vi "TestItemsIndex.vi"(4 "semaphore":T1 caption="信号量", 6 "TestItemIndexIn":i32, 8 "ErrorIn(NoError)":errorcluster, 9 "GuiRef":T2={"StringOut"=refnum, "AbortOnFail"=refnum, "SN"=refnum, "SN_Length"=refnum, "TestResult"=refnum, "CycleTime"=refnum, "ErrorCode"=refnum, "UUTStatus"=refnum, "DataBaseEnable?"=refnum, "DUTModel"=refnum, "FixtureID"=refnum, "OperatorID"=refnum, "SNReady"=refnum, "StopSlot"=refnum, "NextStep"=refnum, "PassYeild"=refnum, "Failed"=refnum, "Passed"=refnum, "Tested"=refnum, "TestItemsCtl"={"StepName"="", "TestEnable"=FALSE, "LoopCount"=0, "StopOnFail"=FALSE, "Index"=0, "TestName"="", "通道"="", "参数"="", "TimeStart"=0}, "ProcessBar"=refnum, "Slot"=enum."Slot1", "Row"=3, "States"=refnum, "TestMode"=refnum, "循环次数-DUT"=refnum, "波形图"=refnum, "产品型号"=refnum, "子面板"=refnum, "测试失败项目"=refnum, "测试结果"=refnum, "DUT"=refnum, "Starttime"=refnum, "SlotReady"=refnum, "版本信息"=refnum, "WIFI_1"=refnum, "WIFI_2"=refnum, "直通率"=refnum, "卡1开卡结果"=refnum, "卡2开卡结果"=refnum}, 11 "Fail项目":string[](array[string])) -> (0 "ErrorOut":errorcluster, 1 "GuiRefOut":T2={"StringOut"=refnum, "AbortOnFail"=refnum, "SN"=refnum, "SN_Length"=refnum, "TestResult"=refnum, "CycleTime"=refnum, "ErrorCode"=refnum, "UUTStatus"=refnum, "DataBaseEnable?"=refnum, "DUTModel"=refnum, "FixtureID"=refnum, "OperatorID"=refnum, "SNReady"=refnum, "StopSlot"=refnum, "NextStep"=refnum, "PassYeild"=refnum, "Failed"=refnum, "Passed"=refnum, "Tested"=refnum, "TestItemsCtl"={"StepName"="", "TestEnable"=FALSE, "LoopCount"=0, "StopOnFail"=FALSE, "Index"=0, "TestName"="", "通道"="", "参数"="", "TimeStart"=0}, "ProcessBar"=refnum, "Slot"=enum."Slot1", "Row"=3, "States"=refnum, "TestMode"=refnum, "循环次数-DUT"=refnum, "波形图"=refnum, "产品型号"=refnum, "子面板"=refnum, "测试失败项目"=refnum, "测试结果"=refnum, "DUT"=refnum, "Starttime"=refnum, "SlotReady"=refnum, "版本信息"=refnum, "WIFI_1"=refnum, "WIFI_2"=refnum, "直通率"=refnum, "卡1开卡结果"=refnum, "卡2开卡结果"=refnum})   [LabVIEW 2013]
uses:
  SysControl/Reference.ctl
  SysControl/TestItemsCTL.ctl
  SysControl/Slot.ctl
  SourceCode/GlobalValue.vi
panel:
  out "Item Names":string[][](array[string])
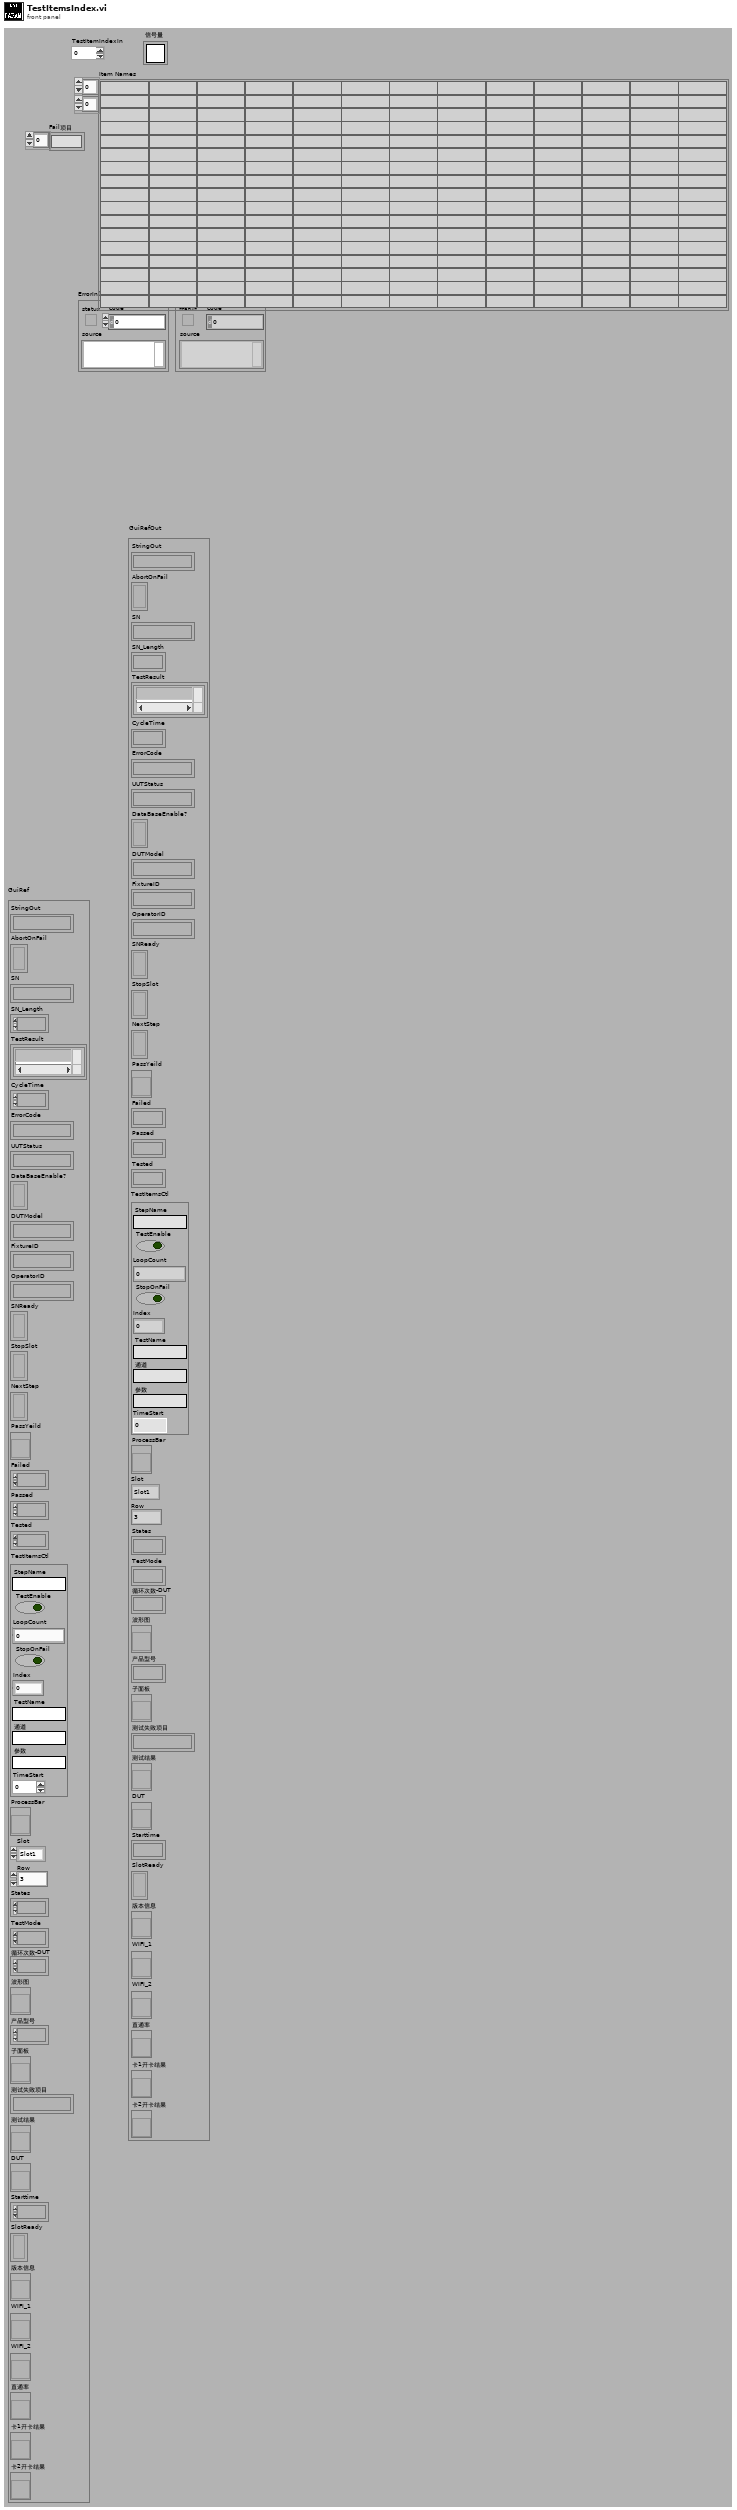
[diagram p1: front panel]
types:
  T1 = typedef "Semaphore RefNum" = refnum<k1>
  T2 = typedef "Reference.ctl" = cluster{"StringOut":refnum<vi>, "AbortOnFail":refnum<vi>, "SN":refnum<vi>, "SN_Length":refnum<vi>, "TestResult":refnum<vi>, "CycleTime":refnum<vi>, "ErrorCode":refnum<vi>, "UUTStatus":refnum<vi>, "DataBaseEnable?":refnum<vi>, "DUTModel":refnum<vi>, "FixtureID":refnum<vi>, "OperatorID":refnum<vi>, "SNReady":refnum<vi>, "StopSlot":refnum<vi>, "NextStep":refnum<vi>, "PassYeild":refnum<vi>, "Failed":refnum<vi>, "Passed":refnum<vi>, "Tested":refnum<vi>, "TestItemsCtl":T3, "ProcessBar":refnum<vi>, "Slot":T4, "Row":u32, "States":refnum<vi>, "TestMode":refnum<vi>, "循环次数-DUT":refnum<vi>, "波形图":refnum<vi>, "产品型号":refnum<vi>, "子面板":refnum<vi>, "测试失败项目":refnum<vi>, "测试结果":refnum<vi>, "DUT":refnum<vi>, "Starttime":refnum<vi>, "SlotReady":refnum<vi>, "版本信息":refnum<vi>, "WIFI_1":refnum<vi>, "WIFI_2":refnum<vi>, "直通率":refnum<vi>, "卡1开卡结果":refnum<vi>, "卡2开卡结果":refnum<vi>}
  T3 = typedef "TestItemsCTL.ctl" = cluster{"StepName":string, "TestEnable":bool, "LoopCount":i32, "StopOnFail":bool, "Index":u32, "TestName":string, "通道":string, "参数":string, "TimeStart":u32}
  T4 = typedef "Slot.ctl" = enum16{"Slot1", "Slot2", "Slot3", "Slot4"}
  T5 = enum16{"Production Mode", "Selection Mode", "Debug Mode", "Loop Mode", "Stop Test"}
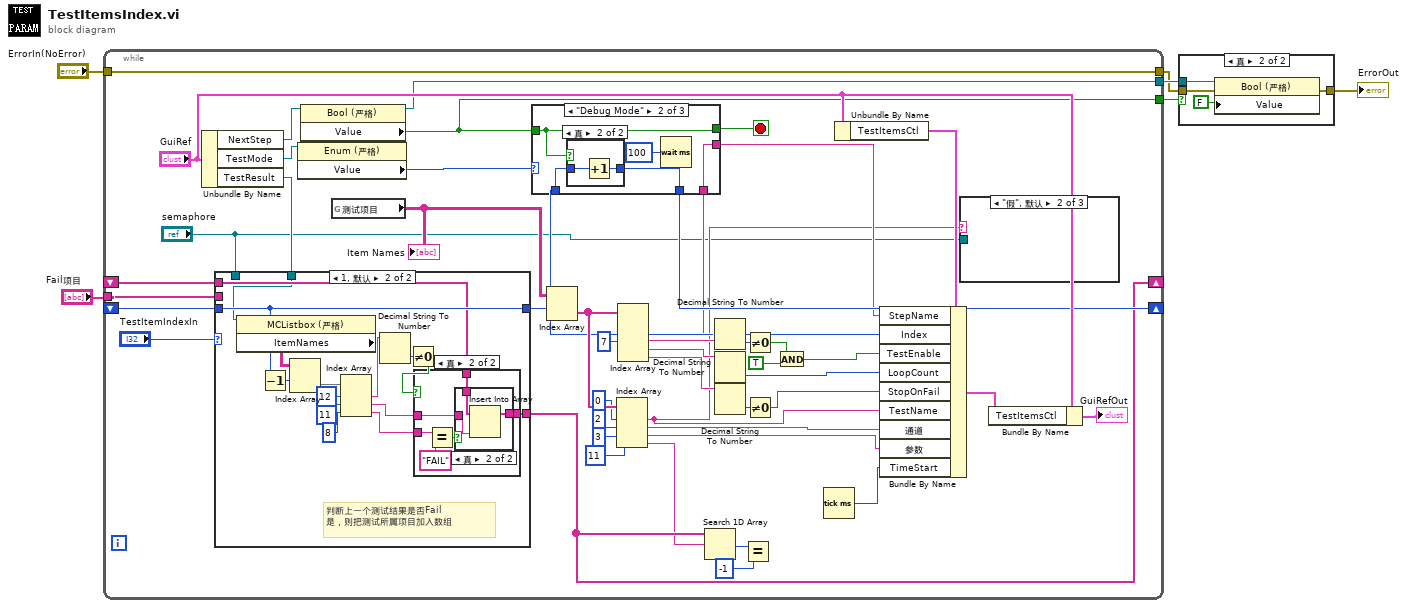
[diagram p0: block diagram]
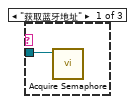
[diagram p3: hidden frame]
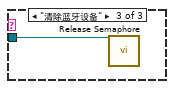
[diagram p4: hidden frame]
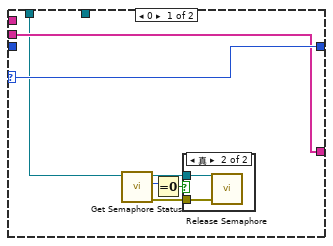
[diagram p5: hidden frame]
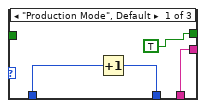
[diagram p9: hidden frame]
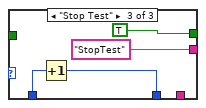
[diagram p11: hidden frame]
diagram:
  n1 = while {
    tunnel: "ErrorIn(NoError)" -> [w41]
    tunnel: [w41] -> w4
    shift-right: [w33] -> _
    shift-left: _ -> [w16]
    tunnel: [w32] -> w5
    tunnel: [w31] -> w3
    shift-right: [w25] -> _
    shift-left: _ -> [w19]
    tunnel: "Fail项目" -> [w20]
    stop <- w10 stop-if-true
    n2 = Unbundle By Name("GuiRef") -> ("NextStep"=w36:refnum<vi>, "TestMode"=w35:refnum<vi>, "TestResult"=w18:refnum<vi>)
    n3 = case shown="1, 默认" "TestItemIndexIn" {
      selector: "TestItemIndexIn" -> [w61 _]
      tunnel: [w61 w76] -> w26
      tunnel: w16 -> [_ w76]
      tunnel: [w60 w75] -> w25
      tunnel: w20 -> [w60 _]
      tunnel: w19 -> [_ w74]
      tunnel: w18 -> [_ w73]
      tunnel: "semaphore" -> [w55 _]
      frame 0 {
        n4 = call <vilib>:"Get Semaphore Status.vi"("semaphore"=w55) -> ("error out"=w57:errorcluster, "# available"=w59:i32, "semaphore out"=w58:T1)  [unwired: 5 in, 3 out]
        n5 = Equal To 0?(x=w59) -> (x = 0?=w56:bool)
        n6 = case shown="真" w56 {
          tunnel: w58 -> [_ w62]
          tunnel: w57 -> [_ w63]
          frame False {
          }
          frame True {
            n7 = call <vilib>:"Release Semaphore.vi"("error in (no error)"=w63, "semaphore"=w62) -> ()  [unwired: 4 in, 2 out]
          }
        }
      }
      frame 1, Default {
        # "判断上一个测试结果是否Fail\n是，则把测试所属项目加入数组"
        n8 = property class="MCListbox (严格)"(reference=w73) -> ("ItemNames"=w72:string[][])  [unwired: 1 in, 2 out]
        n9 = Decrement(x=w76) -> (x-1=w78:i32)
        n10 = Index Array(array=w72, index (row)=w78) -> (element=w77:string[])  [unwired: 1 in]
        n11 = Index Array(array=w77, index #1=12 ("索引"), index #2=11 ("索引"), index #3=8 ("索引")) -> (element #1=w65:string, element #2=w68:string, element #3=w67:string)
        n12 = Decimal String To Number(string=w65) -> (number=w66:i32)  [unwired: 3 out]
        n13 = Not Equal To 0?(x=w66) -> (x != 0?=w64:bool)
        n14 = case shown="真" w64 {
          tunnel: [w79 w83] -> w75
          tunnel: w74 -> [w79 w82]
          tunnel: w68 -> [_ w81]
          tunnel: w67 -> [_ w80]
          frame False {
          }
          frame True {
            n15 = Equal?(x=w80, y="FAIL") -> (x = y?=w85:bool)
            n16 = case shown="真" w85 {
              tunnel: w81 -> [_ w89]
              tunnel: [w86 w88] -> w83
              tunnel: w82 -> [w86 w87]
              frame False {
              }
              frame True {
                n17 = Insert Into Array(array=w87, new element=w89) -> (w88:string[])  [unwired: 1 in]
              }
            }
          }
        }
      }
    }
    n18 = property class="Enum (严格)"(reference=w35) -> ("Value"=w34:T5)  [unwired: 1 in, 2 out]
    n19 = property class="Bool (严格)"(reference=w36) -> (reference out=w32:refnum<vi>, "Value"=w31:bool)  [unwired: 1 in, 1 out]
    n20 = global read "GlobalValue.vi" "测试项目"() -> (w17:string[][])
    "Item Names" <- w17
    n21 = Index Array(array=w17, index (row)=w26) -> (element=w48:string[])  [unwired: 1 in]
    n22 = Index Array(array=w48, index #1=0 ("索引"), index #2=2 ("索引"), index #3=3 ("索引"), index #4=11 ("索引")) -> (element #1=w9:string, element #2=w47:string, element #3=w46:string, element #4=w12:string)
    n23 = Index Array(array=w48, index #3=7 ("index")) -> (element #2=w14:string, element #3=w45:string, element #4=w44:string, element #5=w43:string)  [unwired: 4 in, 1 out]
    n24 = case shown="\"Debug Mode\"" w34 {
      tunnel: w31 -> [_ w95 _]
      tunnel: w26 -> [w93 w98 w105]
      tunnel: [w92 w97 w104] -> w33
      tunnel: [TRUE w95 TRUE] -> w10
      tunnel: w14 -> [w91 w94 _]
      tunnel: [w91 w94 "StopTest" ("element")] -> w11
      frame "Production Mode", Default {
        n25 = Increment(x=w93) -> (x+1=w92:i32)
      }
      frame "Debug Mode" {
        n26 = case shown="真" w95 {
          tunnel: w98 -> [w99 w101]
          tunnel: [w99 w100] -> w97
          frame False {
          }
          frame True {
            n27 = Increment(x=w101) -> (x+1=w100:i32)
          }
        }
        n28 = Wait (ms)(milliseconds to wait=u32 100) -> ()  [unwired: 1 out]
      }
      frame "Stop Test" {
        n29 = Increment(x=w105) -> (x+1=w104:i32)
      }
    }
    n30 = Search 1D Array(1D array=w25, element=w12) -> (index of element=w24:i32)  [unwired: 1 in]
    n31 = Decimal String To Number(string=w45) -> (number=w52:i32)  [unwired: 3 out]
    n32 = Decimal String To Number(string=w44) -> (number=w49:i32)  [unwired: 3 out]
    n33 = Decimal String To Number(string=w43) -> (number=w51:i32)  [unwired: 3 out]
    n34 = Equal?(x=w24, y=-1) -> ()  [unwired: 1 out]
    n35 = Not Equal To 0?(x=w52) -> (x != 0?=w22:bool)
    n36 = Not Equal To 0?(x=w51) -> (x != 0?=w50:bool)
    n37 = And(x=w22, y=TRUE) -> (x .and. y?=w21:bool)
    n38 = Tick Count (ms)() -> (millisecond timer value=w27:u32)
    n39 = Unbundle By Name("GuiRef") -> ("TestItemsCtl"=w38:T3)
    n40 = Bundle By Name(cluster=w38, "StepName"=w11, "Index"=w26, "TestEnable"=w21, "LoopCount"=w49, "StopOnFail"=w50, "TestName"=w9, "通道"=w47, "参数"=w46, "TimeStart"=w27) -> (w40:T3)
    n41 = case shown="\"假\", 默认" w9 {
      tunnel: "semaphore" -> [w53 _ w54]
      frame "获取蓝牙地址" {
        n42 = call <vilib>:"Acquire Semaphore.vi"("semaphore"=w53) -> ()  [unwired: 4 in, 3 out]
      }
      frame "假", Default {
      }
      frame "清除蓝牙设备" {
        n43 = call <vilib>:"Release Semaphore.vi"("semaphore"=w54) -> ()  [unwired: 5 in, 2 out]
      }
    }
    n44 = Bundle By Name(cluster="GuiRef", "TestItemsCtl"=w40) -> (→"GuiRefOut":T2)
  }
  n45 = case shown="真" w3 {
    tunnel: w5 -> [_ w110]
    tunnel: w4 -> [w106 w108]
    tunnel: [w106 w107] -> w1
    frame False {
    }
    frame True {
      n46 = property class="Bool (严格)"(reference=w110, error in=w108, "Value"=FALSE) -> (error out=w107:errorcluster)  [unwired: 1 out]
    }
  }
  "ErrorOut" <- w1
